vi "LinearSystemLoop_Elevator_Pack_Ctrl.vi"(6 "Max Ctrl Out V":dbl=12.0, 7 "Pos Model Std Dev M":dbl=0.04, 8 "Vel Ctrl Tol M/S":dbl=1.0, 9 "Pos Ctrl Tol M":dbl=0.02, 10 "Pos Meas Std Dev M":dbl=0.04, 11 "Vel Model Std Dev M/S":dbl=1.0) -> (3 "LinearSystemLoop_Elevator_Ctrl_Params":T1={"Pos Model Std Dev M"=0.0, "Vel Model Std Dev M/S"=0.0, "Pos Meas Std Dev M"=0.0, "Pos Ctrl Tol M"=0.0, "Vel Ctrl Tol M/S"=0.8, "Max Ctrl Out V"=0.02})   [LabVIEW 2019, in "Trajectory_Library.lvlib"]
uses:
  TypeDef/LINEAR_SYSTEM_LOOP_ELEVATOR_CTRL_PARAMS.CTL
  Trajectory_Library.lvlib
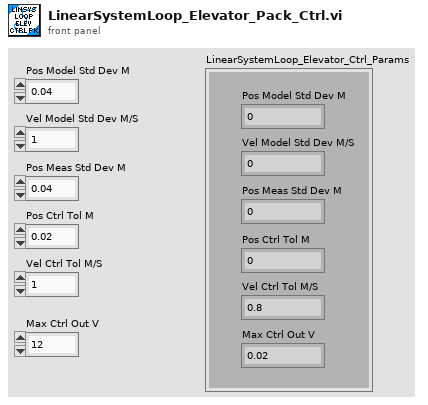
[diagram p1: front panel]
types:
  T1 = typedef "Trajectory_Library.lvlib/LINEAR_SYSTEM_LOOP_ELEVATOR_CTRL_PARAMS.CTL" = cluster{"Pos Model Std Dev M":dbl, "Vel Model Std Dev M/S":dbl, "Pos Meas Std Dev M":dbl, "Pos Ctrl Tol M":dbl, "Vel Ctrl Tol M/S":dbl, "Max Ctrl Out V":dbl}
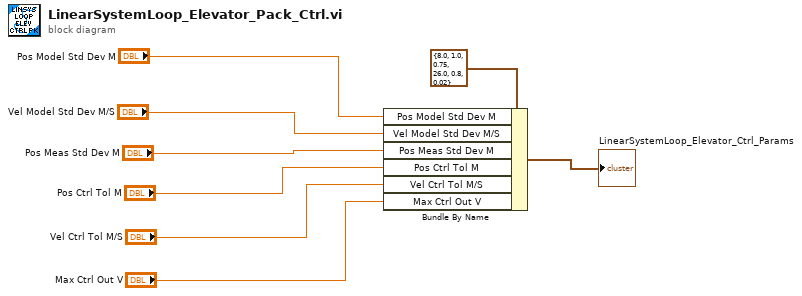
[diagram p0: block diagram]
diagram:
  n1 = Bundle By Name(cluster=T1 {"Pos Model Std Dev M"=8.0, "Vel Model Std Dev M/S"=1.0, "Pos Meas Std Dev M"=0.75, "Pos Ctrl Tol M"=26.0, "Vel Ctrl Tol M/S"=0.8, "Max Ctrl Out V"=0.02} ("DCMotorSim_Model _Params"), "Pos Model Std Dev M"="Pos Model Std Dev M", "Vel Model Std Dev M/S"="Vel Model Std Dev M/S", "Pos Meas Std Dev M"="Pos Meas Std Dev M", "Pos Ctrl Tol M"="Pos Ctrl Tol M", "Vel Ctrl Tol M/S"="Vel Ctrl Tol M/S", "Max Ctrl Out V"="Max Ctrl Out V") -> (→"LinearSystemLoop_Elevator_Ctrl_Params":T1)
